vi "Get Active Cell.vi"(8 "error in (no error)":errorcluster, 9 "Coords":cluster{"Horizontal":i32, "Vertical":i32}, 11 "Multi Listbox Ref In":refnum<vi>) -> (0 "error out":errorcluster, 1 "Active Cell":cluster{"Row":i32, "Column":i32}, 3 "Multi Listbox Ref Out":refnum<vi>, 5 "边界内？":bool)   [LabVIEW 2012]
uses:
  <vilib>/Utility/miscctls.llb/LVRowAndColumnTypeDef.ctl
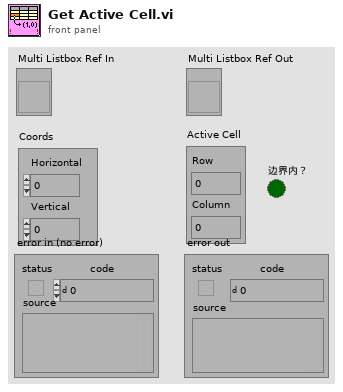
[diagram p1: front panel]
types:
  T1 = typedef "LVRowAndColumnTypeDef.ctl" = cluster{"Row":i32, "Column":i32}
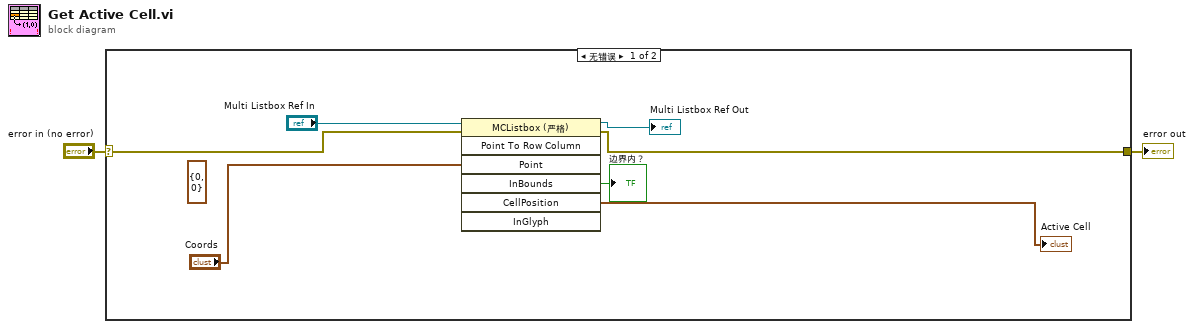
[diagram p0: block diagram]
diagram:
  n1 = case shown="无错误" "error in (no error)" {
    selector: "error in (no error)" -> [w5 w10]
    tunnel: [w4 w10] -> w1
    frame No Error {
      (unwired) T1 {"Row"=0, "Column"=0} ("Active Cell:Active Cell")
      n2 = invoke class="MCListbox (严格)" method="Point To Row Column"(reference="Multi Listbox Ref In", error in=w5, "Point"="Coords") -> (reference out=→"Multi Listbox Ref Out":refnum<vi>, error out=w4:errorcluster, "InBounds"=→"边界内？":bool, "CellPosition"=→"Active Cell":T1)  [unwired: 4 in, 3 out]
    }
    frame Error {
    }
  }
  "error out" <- w1
